vi "SeCrTs-Data Transfer Loop RD.vi"(9 "Message Queue 2":refnum<queue>, 11 "Data FIFO Ref":T1) -> ()   [LabVIEW 2022 SP3]
uses:
  RT Controls/SeCrTs-Data FIFO.ctl
  RT Controls/SeCrTs-DiplayPC comm ctrl.ctl
  <vilib>/Platform/TimedLoop/XDataNode/timing_clust.ctl
  <vilib>/Platform/TimedLoop/XDataNode/nitl_modes.ctl
  <vilib>/Platform/TimedLoop/XDataNode/wakeup.ctl
  RT Support/SeCrTs-RT_Global_R.vi
  <vilib>/platform/TimedLoop/XDataNode/XDataNode.xnode
  <resource>/objmgr/ni.dex.rc
  <vilib>/Platform/TimedLoop/XDataNode/XDNodeRunTimeDep.lvlib
panel:
  out "length":i32
  out "Available Elements for Writing":i32
  out "Buffer Size":i32
  out "x-y 3":i32
  out "Available Elements for Writing":i32
  out "Buffer Size":i32
  out "x-y 2":i32
  out "x-y":u32
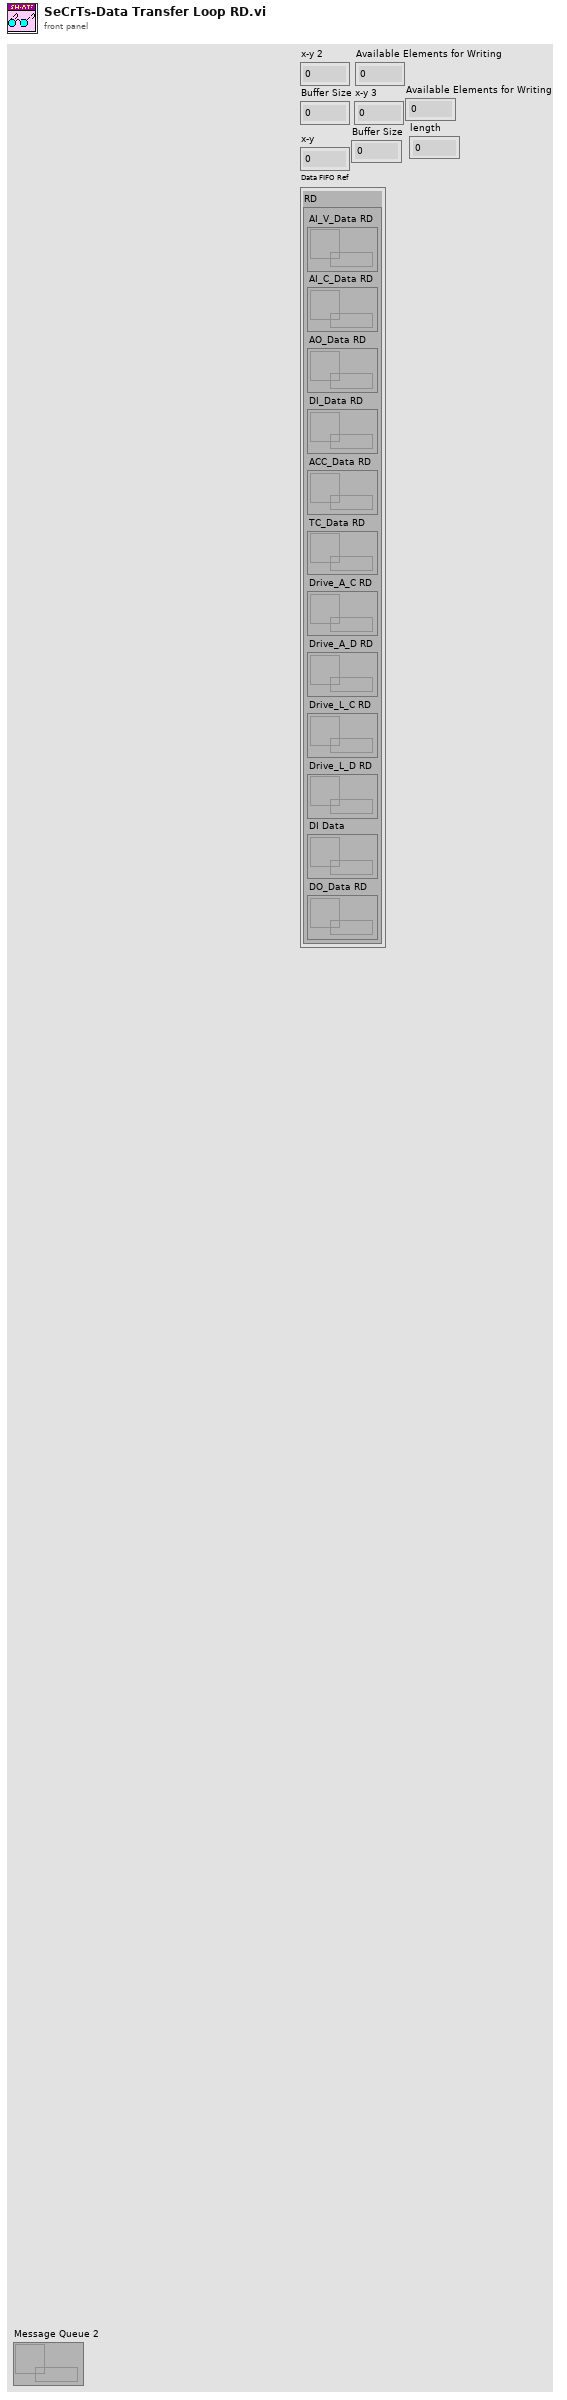
[diagram p1: front panel]
types:
  T1 = typedef "SeCrTs-Data FIFO.ctl" = cluster{"RD":cluster{"AI_V_Data RD":refnum<queue>, "AI_C_Data RD":refnum<queue>, "AO_Data RD":refnum<queue>, "DI_Data RD":refnum<queue>, "ACC_Data RD":refnum<queue>, "TC_Data RD":refnum<queue>, "Drive_A_C RD":refnum<queue>, "Drive_A_D RD":refnum<queue>, "Drive_L_C RD":refnum<queue>, "Drive_L_D RD":refnum<queue>, "DI Data":refnum<queue>, "DO_Data RD":refnum<queue>}}
  T2 = typedef "SeCrTs-DiplayPC comm ctrl.ctl" = enum16{"Initialize", "Listen for UI Writer", "Send RT Data"}
  T3 = typedef "XDNodeRunTimeDep.lvlib/timing_clust.ctl" = cluster{"Expected End [f-1]":u64, "Actual End [f-1]":u64, "Finished Late? [f-1]":bool, "Expected End [i-1]":u64, "Actual End [i-1]":u64, "Finished Late? [i-1]":bool, "Expected Start [i]":u64, "Actual Start [i]":u64, "Expected Start [f]":u64, "Actual Start [f]":u64, "Source Name":string, "Structure Name":string, "Period":i64, "Deadline":i64, "Offset":i64, "Start":i64, "Priority":i32, "Timeout":i32, "Mode":T4, "Wakeup Reason":T5, "Error":errorcluster, "Source Type":string, "Secondary Source Type":string, "Global End Time":u64, "Global Start Time":u64, "Frame Duration":u64, "Iteration Duration":u64, "Assigned CPU":i32, "I/O Scan Engine Mode":u32}
  T4 = typedef "XDNodeRunTimeDep.lvlib/nitl_modes.ctl" = enum32{"No Change", "Process missed periods, maintain original phase", "Discard missed periods, maintain original phase", "Process missed periods, ignore original phase", "Discard missed periods, ignore original phase"}
  T5 = typedef "XDNodeRunTimeDep.lvlib/wakeup.ctl" = enum32{"Normal", "Aborted", "Asynchronous wakeup", "Timing source error", "Timed loop error", "Timeout"}
  T6 = cluster{"Start DAQ":bool, "Stop DAQ":bool, "RT Stop":bool, "RT Exit":bool, "Start Seq":bool}
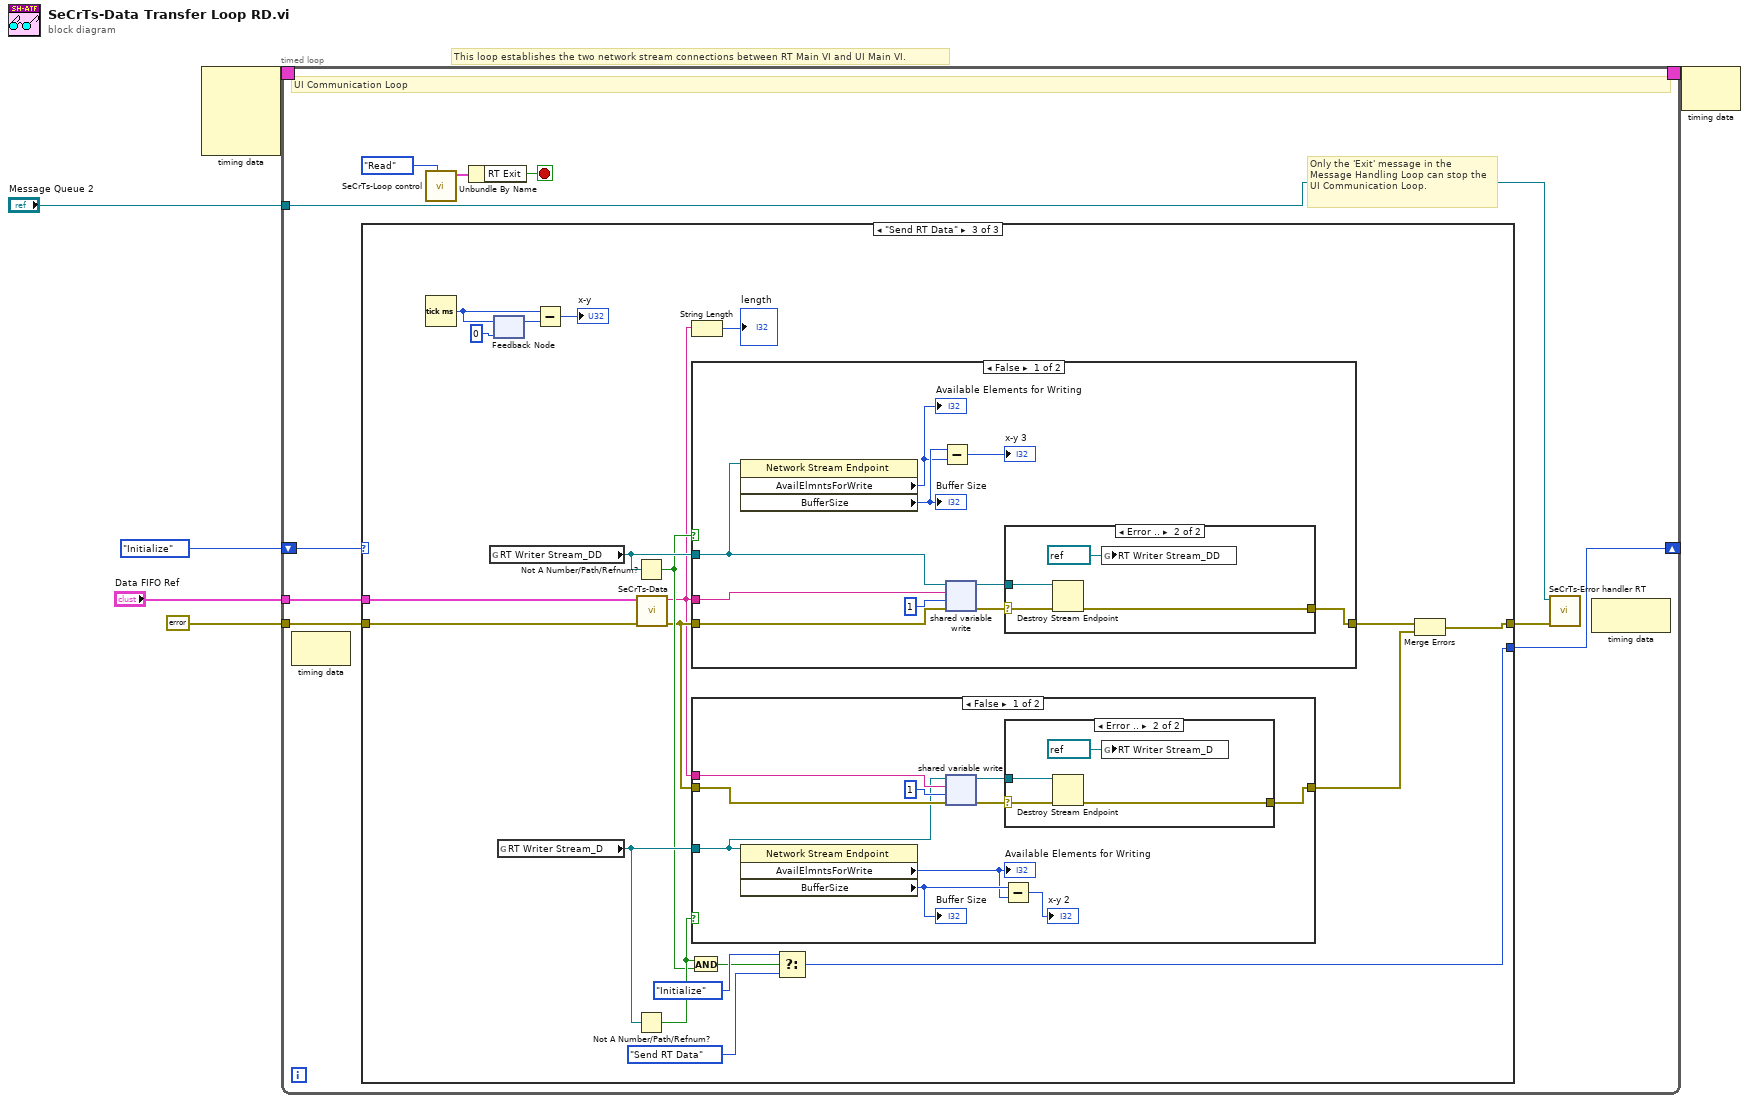
[diagram p0: block diagram]
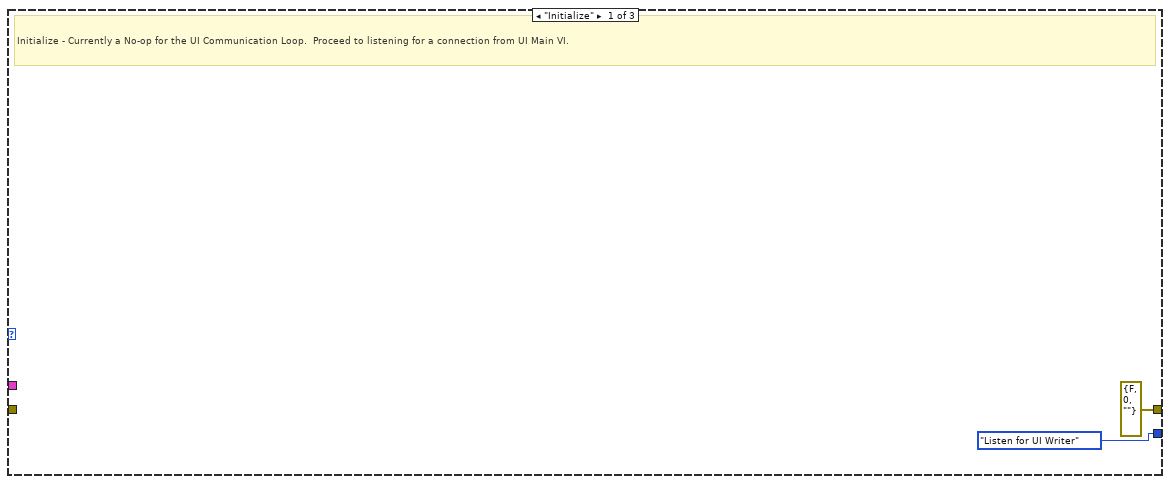
[diagram p2: hidden frame]
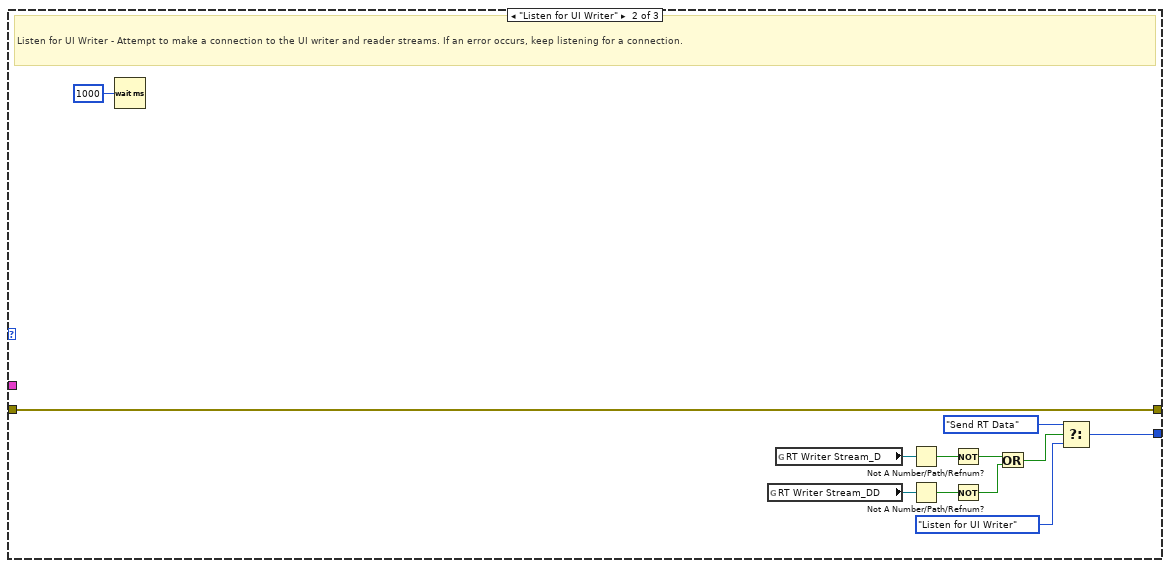
[diagram p3: hidden frame]
diagram:
  # "This loop establishes the two network stream connections between RT Main VI and UI Main VI."
  n1 = node-c288() -> (w2:T3)  [unwired: 4 in]
  n2 = timed-loop {
    shift-right: [w15] -> _
    shift-left: SeCrTs-DiplayPC_comm_ctrl."Initialize" -> [w14]
    tunnel: "Data FIFO Ref" -> [w13]
    tunnel: "Message Queue 2" -> [w9]
    tunnel: errorcluster {"status"=FALSE, "code"=0, "source"=""} ("error in (no error)") -> [w7]
    timing: w2 -> [_]
    timing-out: [_] -> w1
    stop <- w10 stop-if-true
    # "Only the 'Exit' message in the  Message Handling Loop can stop the UI Communication Loop."
    # "UI Communication Loop"
    n3 = node-c288() -> ()  [unwired: 1 in, 1 out]
    n4 = case shown="\"Send RT Data\"" w14 {
      tunnel: [errorcluster {"status"=FALSE, "code"=0, "source"=""} ("error IO") w20 w36] -> w8
      tunnel: [SeCrTs-DiplayPC_comm_ctrl."Listen for UI Writer" w25 w47] -> w15
      tunnel: w13 -> [_ _ w38]
      tunnel: w7 -> [_ w20 w39]
      frame "Initialize" {
        # "Initialize - Currently a No-op for the UI Communication Loop.  Proceed to listening for a connection from UI Main VI."
      }
      frame "Listen for UI Writer" {
        # "Listen for UI Writer - Attempt to make a connection to the UI writer and reader streams. If an error occurs, keep listening for a connection."
        n5 = Wait (ms)(milliseconds to wait=u32 1000) -> ()  [unwired: 1 out]
        n6 = global read "SeCrTs-RT_Global_R.vi" "RT Writer Stream_DD"() -> (w30:refnum<k21>)
        n7 = global read "SeCrTs-RT_Global_R.vi" "RT Writer Stream_D"() -> (w31:refnum<k21>)
        n8 = Not A Number/Path/Refnum?(number/path/refnum=w31) -> (NaN/Path/Refnum?=w29:bool)
        n9 = Not A Number/Path/Refnum?(number/path/refnum=w30) -> (NaN/Path/Refnum?=w28:bool)
        n10 = Not(x=w29) -> (.not. x?=w27:bool)
        n11 = Not(x=w28) -> (.not. x?=w26:bool)
        n12 = Or(x=w27, y=w26) -> (x .or. y?=w22:bool)
        n13 = Select(t=SeCrTs-DiplayPC_comm_ctrl."Send RT Data", s=w22, f=SeCrTs-DiplayPC_comm_ctrl."Listen for UI Writer") -> (s? t:f=w25:T2)
      }
      frame "Send RT Data" {
        n14 = Tick Count (ms)() -> (millisecond timer value=w44:u32)
        n15 = global read "SeCrTs-RT_Global_R.vi" "RT Writer Stream_DD"() -> (w45:refnum<k21>)
        n16 = feedback-in #1(w44) -> ()
        n17 = feedback #1(u32 0 ("millisecond timer value")) -> (w43:u32)
        n18 = global read "SeCrTs-RT_Global_R.vi" "RT Writer Stream_D"() -> (w51:refnum<k21>)
        n19 = Subtract(x=w44, y=w43) -> (x-y=→"x-y":u32)
        n20 = Not A Number/Path/Refnum?(number/path/refnum=w45) -> (NaN/Path/Refnum?=w40:bool)
        n21 = Not A Number/Path/Refnum?(number/path/refnum=w51) -> (NaN/Path/Refnum?=w46:bool)
        n22 = call "SeCrTs-Data.vi"("error in (no error)"=w39, "Data FIFO Ref"=w38) -> ("error out"=w34:errorcluster, "data"=w33:string)  [unwired: 8 in]
        n23 = And(x=w46, y=w40) -> (x .and. y?=w48:bool)
        n24 = String Length(string=w33) -> (length=→"length":i32)
        n25 = case shown="False" w40 {
          tunnel: w45 -> [w52 _]
          tunnel: w34 -> [w59 w67]
          tunnel: [w58 w67] -> w41
          tunnel: w33 -> [w57 _]
          frame False {
            n26 = property class="Network Stream Endpoint"(reference=w52) -> ("AvailElmntsForWrite"=w53:i32, "BufferSize"=w54:i32)  [unwired: 1 in, 2 out]
            "Buffer Size" <- w54
            "Available Elements for Writing" <- w53
            n27 = Subtract(x=w54, y=w53) -> (x-y=→"x-y 3":i32)
            n28 = shared-variable-write(w52, w59, w57, 1 ("timeout ms (-1)")) -> (w60:refnum<k21>, w61:errorcluster)  [unwired: 1 out]
            n29 = case shown="Error .." w61 {
              selector: w61 -> [w62 w65]
              tunnel: w60 -> [_ w66]
              tunnel: [w62 w63] -> w58
              frame No Error {
              }
              frame Error {
                n30 = Destroy Stream Endpoint(8:w65, 11:w66) -> (0:w63:errorcluster)
                n31 = global write "SeCrTs-RT_Global_R.vi" "RT Writer Stream_DD"(refnum<k21> refnum ("RT Writer Stream_DD")) -> ()
              }
            }
          }
          frame True {
          }
        }
        n32 = case shown="False" w46 {
          tunnel: w51 -> [w71 _]
          tunnel: w34 -> [w74 w83]
          tunnel: [w75 w83] -> w35
          tunnel: w33 -> [w73 _]
          frame False {
            n33 = property class="Network Stream Endpoint"(reference=w71) -> ("AvailElmntsForWrite"=w68:i32, "BufferSize"=w69:i32)  [unwired: 1 in, 2 out]
            "Buffer Size" <- w69
            "Available Elements for Writing" <- w68
            n34 = shared-variable-write(w71, w74, w73, 1 ("timeout ms (-1)")) -> (w76:refnum<k21>, w77:errorcluster)  [unwired: 1 out]
            n35 = Subtract(x=w69, y=w68) -> (x-y=→"x-y 2":i32)
            n36 = case shown="Error .." w77 {
              selector: w77 -> [w78 w81]
              tunnel: w76 -> [_ w82]
              tunnel: [w78 w79] -> w75
              frame No Error {
              }
              frame Error {
                n37 = Destroy Stream Endpoint(8:w81, 11:w82) -> (0:w79:errorcluster)
                n38 = global write "SeCrTs-RT_Global_R.vi" "RT Writer Stream_D"(refnum<k21> refnum ("RT Writer Stream_DD")) -> ()
              }
            }
          }
          frame True {
          }
        }
        n39 = Select(t=SeCrTs-DiplayPC_comm_ctrl."Initialize", s=w48, f=SeCrTs-DiplayPC_comm_ctrl."Send RT Data") -> (s? t:f=w47:T2)
        n40 = Merge Errors(w41, w35) -> (w36:errorcluster)
      }
    }
    n41 = call "SeCrTs-Loop control.vi"("Action"=enum16{"Init", "Write", "Read"}."Read") -> ("Loop Control out"=w12:T6)  [unwired: 9 in, 1 out]
    n42 = Unbundle By Name(w12) -> ("RT Exit"=w10:bool)
    n43 = call "SeCrTs-Error handler RT.vi"("error in"=w8, "Message Queue"=w9) -> ()  [unwired: 8 in, 2 out]
    n44 = node-c288() -> ()  [unwired: 1 in, 1 out]
  }
  n45 = node-c288(w1) -> ()  [unwired: 1 out]
